vi "CSM - Interface Browser.vi"(10 "Init State (\"Macro: Initialize\")":string="Macro: Initialize") -> ()   [LabVIEW 2017]
uses:
  <vilib>/Utility/miscctls.llb/LVRectTypeDef.ctl
  Communicable State Machine.lvlib
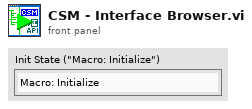
[diagram p1: front panel]
types:
  T1 = typedef "LVRectTypeDef.ctl" = cluster{"Left":i16, "Top":i16, "Right":i16, "Bottom":i16}
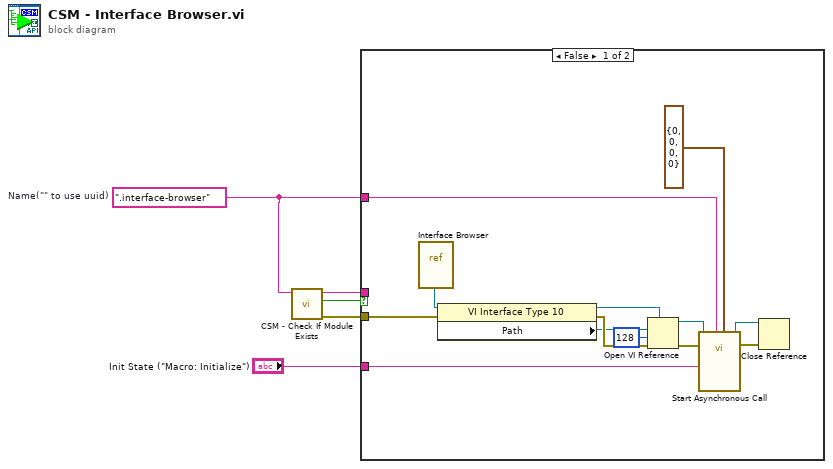
[diagram p0: block diagram]
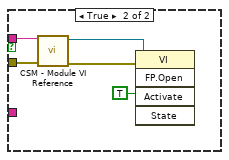
[diagram p2: hidden frame]
diagram:
  w5 = ".interface-browser"  # Name("" to use uuid)
  n1 = call "CSM - Check If Module Exists.vi"("CSM Name"=w5) -> ("error out"=w4:errorcluster, "Exist?"=w3:bool, "CSM Name (Dup)"=w2:string)  [unwired: 8 in]
  n2 = case shown="False" w3 {
    tunnel: w5 -> [w8 _]
    tunnel: w4 -> [w7 w22]
    tunnel: w2 -> [_ w23]
    tunnel: "Init State (\"Macro: Initialize\")" -> [w6 _]
    frame False {
      n3 = vi-ref "Interface Browser.vi"() -> (w11:refnum<vi>)
      n4 = property class="VI Interface Type 10"(reference=w11, error in=w7) -> (reference out=w15:refnum<vi>, error out=w13:errorcluster, "Path"=w12:path)
      n5 = Open VI Reference(type specifier VI Refnum (for type only)=w15, vi path=w12, options=128, error in (no error)=w13) -> (vi reference=w14:refnum<vi>, error out=w10:errorcluster)  [unwired: 2 in]
      n6 = call-by-ref "Start Asynchronous Call"(reference=w14, error in=w10, "Caller Window Bounds"=T1 {"Left"=0, "Top"=0, "Right"=0, "Bottom"=0}, "Name(\"\" to use uuid)"=w8, "Init State(\"Macro: Initialize\")"=w6) -> (reference out=w17:refnum<vi>, error out=w16:errorcluster)  [unwired: 9 in]
      n7 = Close Reference(reference=w17, error in (no error)=w16) -> ()  [unwired: 1 out]
    }
    frame True {
      n8 = call "CSM - Module VI Reference.vi"("error in (no error)"=w22, "CSM Name"=w23) -> ("error out"=w21:errorcluster, "CSM Module VIRef"=w20:refnum<vi>)  [unwired: 8 in]
      n9 = invoke class="VI" method="FP.Open"(reference=w20, error in=w21, "Activate"=TRUE ("Activate?")) -> ()  [unwired: 2 in, 5 out]
    }
  }
